vi "ReadPressureSensor.vi"(8 "error in (no error)":errorcluster, 9 "BMP180 Config Options":T2 {"I2C"."Slave Address" format="%.0x"; "Cal Coefs"."MD"."Val:" format="%04x"; "Cal Coefs"."MD"."Addr:" format="%02x"; "Cal Coefs"."MC"."Val:" format="%04x"; "Cal Coefs"."MC"."Addr:" format="%02x"; "Cal Coefs"."MB"."Val:" format="%04x"; "Cal Coefs"."MB"."Addr:" format="%02x"; "Cal Coefs"."B2"."Val:" format="%04x"; "Cal Coefs"."B2"."Addr:" format="%02x"; "Cal Coefs"."B1"."Val:" format="%04x"; "Cal Coefs"."B1"."Addr:" format="%02x"; "Cal Coefs"."AC6"."Val:" format="%04x"; "Cal Coefs"."AC6"."Addr:" format="%02x"; "Cal Coefs"."AC5"."Val:" format="%04x"; "Cal Coefs"."AC5"."Addr:" format="%02x"; "Cal Coefs"."AC4"."Val:" format="%04x"; "Cal Coefs"."AC4"."Addr:" format="%02x"; "Cal Coefs"."AC3"."Val:" format="%04x"; "Cal Coefs"."AC3"."Addr:" format="%02x"; "Cal Coefs"."AC2"."Val:" format="%04x"; "Cal Coefs"."AC2"."Addr:" format="%02x"; "Cal Coefs"."AC1"."Val:" format="%04x"; "Cal Coefs"."AC1"."Addr:" format="%02x"}) -> (0 "error out":errorcluster, 1 "BMP180 Config":T2 {"I2C"."Slave Address" format="%.0x"; "Cal Coefs"."MD"."Val:" format="%04x"; "Cal Coefs"."MD"."Addr:" format="%02x"; "Cal Coefs"."MC"."Val:" format="%04x"; "Cal Coefs"."MC"."Addr:" format="%02x"; "Cal Coefs"."MB"."Val:" format="%04x"; "Cal Coefs"."MB"."Addr:" format="%02x"; "Cal Coefs"."B2"."Val:" format="%04x"; "Cal Coefs"."B2"."Addr:" format="%02x"; "Cal Coefs"."B1"."Val:" format="%04x"; "Cal Coefs"."B1"."Addr:" format="%02x"; "Cal Coefs"."AC6"."Val:" format="%04x"; "Cal Coefs"."AC6"."Addr:" format="%02x"; "Cal Coefs"."AC5"."Val:" format="%04x"; "Cal Coefs"."AC5"."Addr:" format="%02x"; "Cal Coefs"."AC4"."Val:" format="%04x"; "Cal Coefs"."AC4"."Addr:" format="%02x"; "Cal Coefs"."AC3"."Val:" format="%04x"; "Cal Coefs"."AC3"."Addr:" format="%02x"; "Cal Coefs"."AC2"."Val:" format="%04x"; "Cal Coefs"."AC2"."Addr:" format="%02x"; "Cal Coefs"."AC1"."Val:" format="%04x"; "Cal Coefs"."AC1"."Addr:" format="%02x"}, 2 "Pressure Reading":T1)   [LabVIEW 2017]
uses:
  Sensors/Pressure Sensor - BMP180/BMP180 Config Options.ctl
  Type Defs/pressureReading.ctl
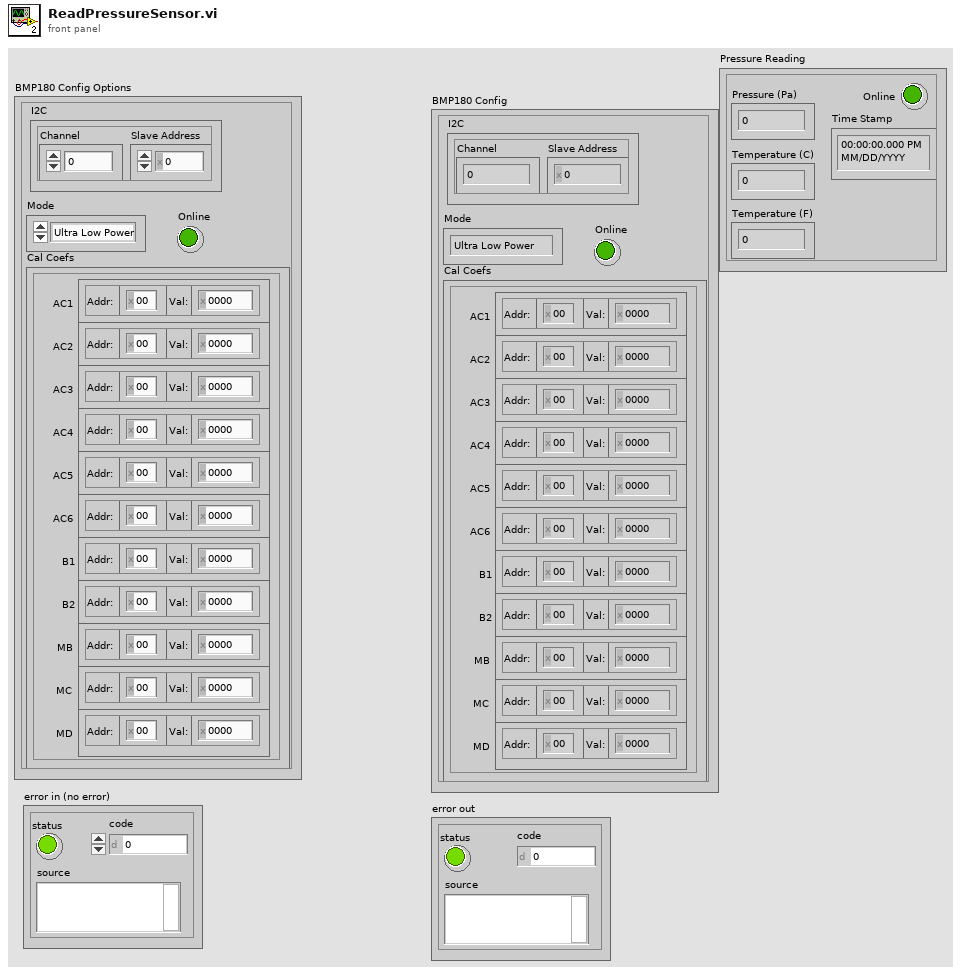
[diagram p1: front panel]
types:
  T1 = typedef "pressureReading.ctl" = cluster{"Time Stamp":timestamp, "Online":bool, "Temperature (C)":dbl, "Pressure (Pa)":dbl, "Temperature (F)":dbl}
  T2 = typedef "BMP180 Config Options.ctl" = cluster{"I2C":cluster{"Slave Address":u8, "Channel":u8}, "Mode":enum8{"Ultra Low Power", "Standard", "High Resolution", "Ultra High Resolution"}, "Cal Coefs":cluster{"AC1":cluster{"Addr:":u8, "Val:":u16}, "AC2":cluster{"Addr:":u8, "Val:":u16}, "AC3":cluster{"Addr:":u8, "Val:":u16}, "AC4":cluster{"Addr:":u8, "Val:":u16}, "AC5":cluster{"Addr:":u8, "Val:":u16}, "AC6":cluster{"Addr:":u8, "Val:":u16}, "B1":cluster{"Addr:":u8, "Val:":u16}, "B2":cluster{"Addr:":u8, "Val:":u16}, "MB":cluster{"Addr:":u8, "Val:":u16}, "MC":cluster{"Addr:":u8, "Val:":u16}, "MD":cluster{"Addr:":u8, "Val:":u16}}, "Online":bool}
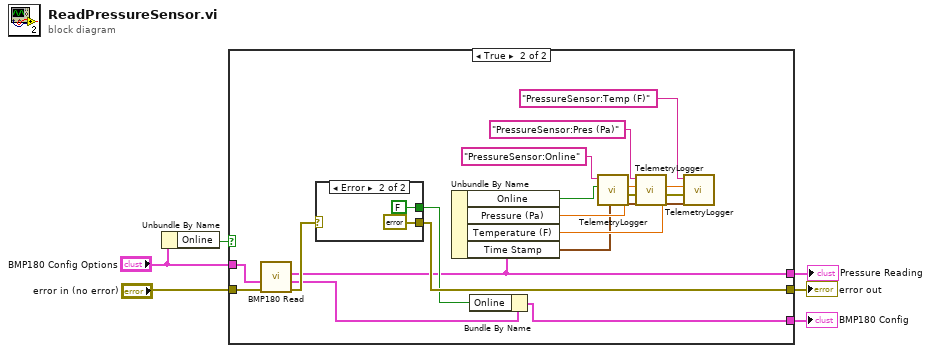
[diagram p0: block diagram]
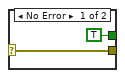
[diagram p3: hidden frame]
diagram:
  n1 = Unbundle By Name("BMP180 Config Options") -> ("Online"=w2:bool)
  n2 = case shown="True" w2 {
    tunnel: "error in (no error)" -> [w7 w25]
    tunnel: [w7 w20] -> w5
    tunnel: "BMP180 Config Options" -> [w8 w17]
    tunnel: [w8 w18] -> w4
    tunnel: [_ w15] -> w1
    frame False {
    }
    frame True {
      n3 = call "BMP180 Read.vi"("error in (no error)"=w25, "BMP180 Config"=w17) -> ("error out"=w21:errorcluster, "BMP180 Config"=w16:T2, "Pressure Reading"=w15:T1)  [unwired: 6 in, 1 out]
      n4 = case shown="Error" w21 {
        selector: w21 -> [w27 _]
        tunnel: [w27 errorcluster {"status"=FALSE, "code"=0, "source"=""} ("error IO")] -> w20
        tunnel: [TRUE FALSE] -> w19
        frame No Error {
        }
        frame Error {
        }
      }
      n5 = Unbundle By Name(w15) -> ("Online"=w14:bool, "Pressure (Pa)"=w13:dbl, "Temperature (F)"=w12:dbl, "Time Stamp"=w11:timestamp)
      n6 = Bundle By Name(cluster=w16, "Online"=w19) -> (w18:T2)
      n7 = call "TelemetryLogger.vi"("Time Stamp"=w11, "Data"=w14, "Sensor:Reading"="PressureSensor:Online") -> ("Error Out"=w10:errorcluster)  [unwired: 8 in]
      n8 = call "TelemetryLogger.vi"("Time Stamp"=w11, "Error In"=w10, "Data"=w13, "Sensor:Reading"="PressureSensor:Pres (Pa)") -> ("Error Out"=w9:errorcluster)  [unwired: 7 in]
      n9 = call "TelemetryLogger.vi"("Time Stamp"=w11, "Error In"=w9, "Data"=w12, "Sensor:Reading"="PressureSensor:Temp (F)") -> ()  [unwired: 7 in, 1 out]
    }
  }
  "error out" <- w5
  "BMP180 Config" <- w4
  "Pressure Reading" <- w1
